vi "_TCP-IP_Q_Bridge._Test_Sta.vi"() -> ()   [LabVIEW 2024, in "EQMF.lvlib" / "TCP-IP.lvlib"]
uses:
  TCP-IP.lvlib
  Mgr/TCP-IP Mgr.Config.ctl
  Queues/Queue Utils.lvlib
panel:
  in  "Notification":bool
  out "Con Status":bool
  out "Rcv Cluster":T1={"Enum"=enum."B", "Numeric"=6.0, "Boolean"=TRUE, "String"="ABBCC"}
  in  "Cluster":T1={"Enum"=enum."B", "Numeric"=6.0, "Boolean"=TRUE, "String"="ABBCC"}
  in  "Send Cluster":bool
  in  "Config":T2={"IP"="127.0.0.1", "Port"=8500, "Listener"=TRUE, "Enable"=FALSE}
  out "Connected":bool
  in  "Exit":bool
  out "Rcv Bool":bool
  in  "Send Str":bool
  out "Rcv String":string
  in  "String":string
  in  "Data":bool
  in  "Send Data":bool
  # "Child"
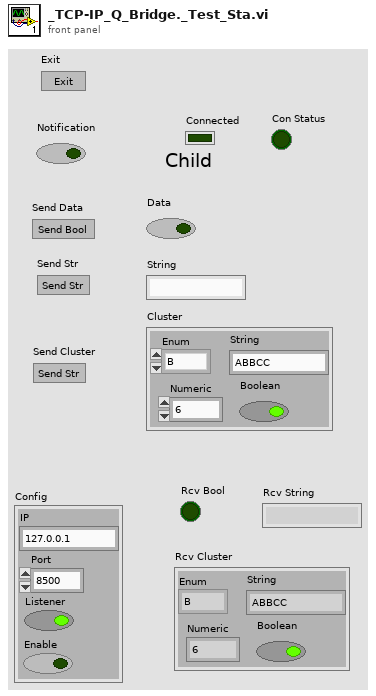
[diagram p1: front panel]
types:
  T1 = cluster{"Enum":enum16{"A", "B", "C"}, "Numeric":dbl, "Boolean":bool, "String":string}
  T2 = typedef "EQMF.lvlib/TCP-IP.lvlib/TCP-IP Mgr.Config.ctl" = cluster{"IP":string, "Port":u16, "Listener":bool, "Enable":bool}
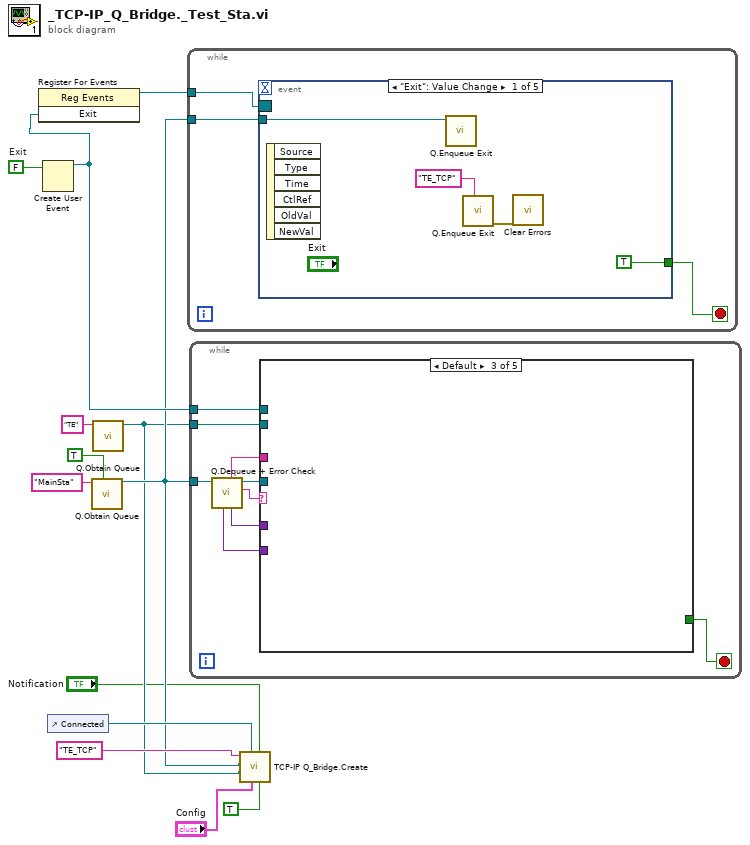
[diagram p0: block diagram]
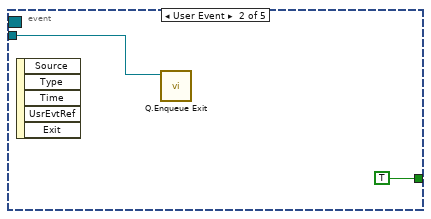
[diagram p2: hidden frame]
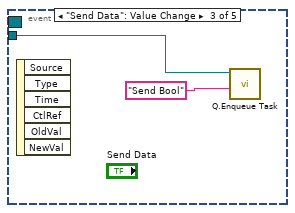
[diagram p3: hidden frame]
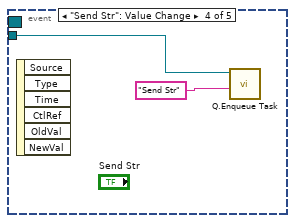
[diagram p4: hidden frame]
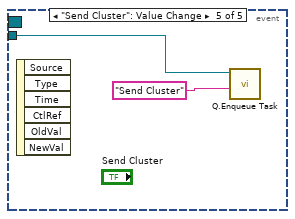
[diagram p5: hidden frame]
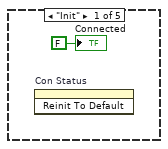
[diagram p6: hidden frame]
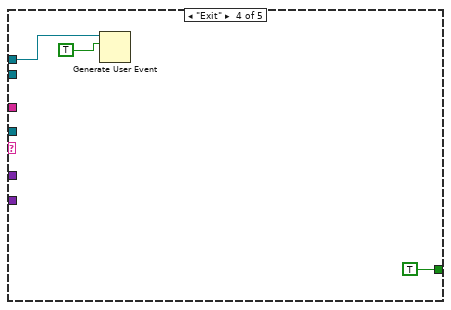
[diagram p8: hidden frame]
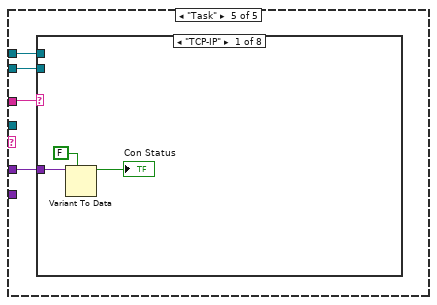
[diagram p9: hidden frame]
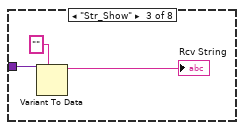
[diagram p11: hidden frame]
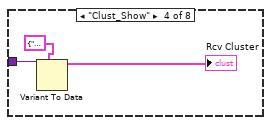
[diagram p12: hidden frame]
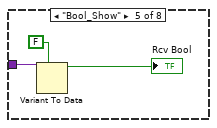
[diagram p13: hidden frame]
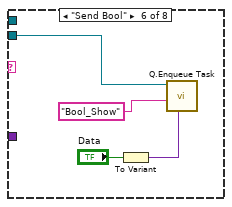
[diagram p14: hidden frame]
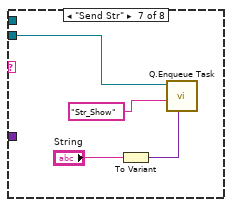
[diagram p15: hidden frame]
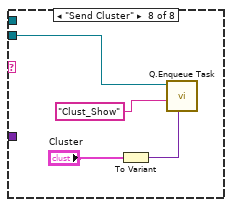
[diagram p16: hidden frame]
diagram:
  w11 = FALSE  # Exit
  n1 = Create User Event(user event datatype=w11) -> (user event=w9:refnum<user-event>)  [unwired: 1 in, 1 out]
  n2 = register-events(w9) -> (reference out=w10:refnum<event-registration>)  [unwired: 2 in, 1 out]
  n3 = control-ref of="Connected"() -> (w8:refnum<vi>)
  n4 = call "Q.Obtain Queue.vi"("Enqueue Init"=TRUE, "Q Name"="MainSta") -> ("Q Out"=w6:refnum<queue>)  [unwired: 7 in, 2 out]
  n5 = call "Q.Obtain Queue.vi"("Q Name"="TE") -> ("Q Out"=w5:refnum<queue>)  [unwired: 8 in, 2 out]
  n6 = while {
    tunnel: w6 -> [w16]
    tunnel: w10 -> [w14]
    stop <- w15 stop-if-true
    n7 = event shown="[0] \"Exit\": Value Change" {
      selector: w14 -> [_ _ _ _ _]
      dyn-events: _ -> [_ _ _ _ _]
      timeout: _ -> [_ _ _ _ _]
      tunnel: w16 -> [w20 w22 w24 w26 w28]
      tunnel: [TRUE TRUE _ _ _] -> w15
      event "Exit": Value Change {
        n8 = event-data() -> ()  [unwired: 1 in, 6 out]
        n9 = call "Q.Enqueue Exit.vi"("Q In"=w20) -> ()  [unwired: 9 in, 2 out]
        n10 = call "Q.Enqueue Exit.vi"("Q Name"="TE_TCP") -> ("error out"=w18:errorcluster)  [unwired: 9 in, 1 out]
        n11 = call <vilib>:"Clear Errors.vi"("error in (no error)"=w18) -> ()  [unwired: 5 in, 2 out]
      }
      event User Event {
        n12 = event-data() -> ()  [unwired: 1 in, 5 out]
        n13 = call "Q.Enqueue Exit.vi"("Q In"=w22) -> ()  [unwired: 9 in, 2 out]
      }
      event "Send Data": Value Change {
        n14 = event-data() -> ()  [unwired: 1 in, 6 out]
        n15 = call "Q.Enqueue Task.vi"("Task Name"="Send Bool", "Q In"=w24) -> ()  [unwired: 8 in, 2 out]
      }
      event "Send Str": Value Change {
        n16 = event-data() -> ()  [unwired: 1 in, 6 out]
        n17 = call "Q.Enqueue Task.vi"("Task Name"="Send Str", "Q In"=w26) -> ()  [unwired: 8 in, 2 out]
      }
      event "Send Cluster": Value Change {
        n18 = event-data() -> ()  [unwired: 1 in, 6 out]
        n19 = call "Q.Enqueue Task.vi"("Task Name"="Send Cluster", "Q In"=w28) -> ()  [unwired: 8 in, 2 out]
      }
    }
  }
  n20 = while {
    tunnel: w6 -> [w36]
    tunnel: w5 -> [w30]
    tunnel: w9 -> [w29]
    stop <- w31 stop-if-true
    n21 = call "Q.Dequeue + Error Check.vi"("Q In"=w36) -> ("Cmd"=w37:string, "Q Out"=w35:refnum<queue>, "Data1"=w33:variant, "Sub"=w34:string, "Data2"=w32:variant)  [unwired: 5 in, 1 out]
    n22 = case shown="Default" w37 {
      tunnel: w35 -> [_ _ _ _ _]
      tunnel: w34 -> [_ _ _ _ w45]
      tunnel: w33 -> [_ _ _ _ w44]
      tunnel: w32 -> [_ _ _ _ _]
      tunnel: [_ _ _ TRUE _] -> w31
      tunnel: w30 -> [_ _ _ _ w43]
      tunnel: w29 -> [_ _ _ w39 w42]
      frame "Init" {
        n23 = invoke on="Con Status" class="Bool (strict)" method="Reinit To Default"() -> ()  [unwired: 3 in, 3 out]
        "Connected" <- FALSE ("Connected")
      }
      frame "Reset" {
      }
      frame Default {
      }
      frame "Exit" {
        n24 = Generate User Event(user event=w39, event data cluster=TRUE) -> ()  [unwired: 2 in, 2 out]
      }
      frame "Task" {
        n25 = case shown="\"TCP-IP\"" w45 {
          tunnel: w44 -> [w48 _ w51 w54 w57 _ _ _]
          tunnel: w43 -> [_ _ _ _ _ w61 w65 w69]
          tunnel: w42 -> [_ _ _ _ _ _ _ _]
          frame "TCP-IP" {
            n26 = Variant To Data(type=FALSE, Variant=w48) -> (data=→"Con Status":bool)  [unwired: 1 in, 1 out]
          }
          frame Default {
          }
          frame "Str_Show" {
            n27 = Variant To Data(type="", Variant=w51) -> (data=→"Rcv String":string)  [unwired: 1 in, 1 out]
          }
          frame "Clust_Show" {
            n28 = Variant To Data(type=T1 {"Enum"=enum."B", "Numeric"=6.0, "Boolean"=TRUE, "String"="ABBCC"} ("Rcv Cluster"), Variant=w54) -> (data=→"Rcv Cluster":T1)  [unwired: 1 in, 1 out]
          }
          frame "Bool_Show" {
            n29 = Variant To Data(type=FALSE, Variant=w57) -> (data=→"Rcv Bool":bool)  [unwired: 1 in, 1 out]
          }
          frame "Send Bool" {
            n30 = To Variant(anything="Data") -> (Variant=w58:variant)
            n31 = call "Q.Enqueue Task.vi"("Data1"=w58, "Task Name"="Bool_Show", "Q In"=w61) -> ()  [unwired: 7 in, 2 out]
          }
          frame "Send Str" {
            n32 = To Variant(anything="String") -> (Variant=w63:variant)
            n33 = call "Q.Enqueue Task.vi"("Data1"=w63, "Task Name"="Str_Show", "Q In"=w65) -> ()  [unwired: 7 in, 2 out]
          }
          frame "Send Cluster" {
            n34 = To Variant(anything="Cluster") -> (Variant=w67:variant)
            n35 = call "Q.Enqueue Task.vi"("Data1"=w67, "Task Name"="Clust_Show", "Q In"=w69) -> ()  [unwired: 7 in, 2 out]
          }
        }
      }
    }
  }
  n36 = call "TCP-IP Q_Bridge.Create.vi"("Auto Exit"=TRUE, "Notification"="Notification", "Config"="Config", "StatusCtrlRef"=w8, "Q_DataOut"=w5, "Q_DataIn"=w6, "Control Q Name"="TE_TCP" ("Q Name")) -> ()  [unwired: 3 in, 2 out]
